vi "Compiled Get Sim Device Settings.vi"(8 "error in (no error)":errorcluster, 9 "Cluster":refnum<k21>, 11 "Addon Ref":T1 format="%.0x") -> (0 "error out":errorcluster, 1 "Async Refs":T2(array[cluster]) {"VS Refs" format="%.0x"}, 2 "Settings":T3[](array[typedef]) {"DTCs"."DM1.Ref"."Data Reference" format="%.0x"; "DTCs"."DM1.Enable.Ref"."Data Reference" format="%.0x"; "DTCs"."DM2.Ref"."Data Reference" format="%.0x"; "DTCs"."DM2.Enable.Ref"."Data Reference" format="%.0x"; "Data"."Outgoing"."Trigger.Refs"."Data Reference" format="%.0x"; "Data"."Outgoing"."Disable.Refs"."Data Reference" format="%.0x"; "Data"."Outgoing"."Data.Refs"."Data Reference" format="%.0x"; "Data"."Incoming"."Timing.Refs"."Data Reference" format="%.0x"; "Data"."Incoming"."Data.Refs"."Data Reference" format="%.0x"; "Network"."Name" format="%.0x"}, 3 "Addon Ref out":T1 format="%.0x")   [LabVIEW 2023, in "J1939 Addon System Explorer.lvlib"]
uses:
  J1939 Addon System Explorer.lvlib
  <vilib>/NI VeriStand/Custom Device API/Custom Device Item Ref.ctl
  Addon Shared/Types/Complied Simulated Device Settings.ctl
  Addon Shared/Types/Monitor Settings.ctl
  Addon Shared/Types/Device Settings.ctl
  Addon Shared/Types/Incoming Settings.ctl
  Addon Shared/Types/Incoming Frame Settings.ctl
  <vilib>/NI VeriStand/Custom Device API/Block Data Reference.ctl
  <vilib>/NI VeriStand/Custom Device API/Data Reference.ctl
  Addon Shared/Types/Outgoing Settings.ctl
  Addon Shared/Types/Outgoing Frame Settings.ctl
  Addon Shared/Types/Outgoing Event Trigger Types.ctl
  SubModules/Frame-Protection-Support/Source/Shared/Types/Exported Frame Settings.ctl
  SubModules/Frame-Protection-Support/Source/Shared/Types/Exported Frame Type.ctl
  SubModules/Frame-Protection-Support/Source/Shared/Types/Exported Protection Settings.ctl
  SubModules/Frame-Protection-Support/Source/Shared/Types/Protection Type.ctl
  SubModules/Frame-Protection-Support/Source/Shared/Types/XNET Signal Configuration.ctl
  SubModules/Frame-Protection-Support/Source/Shared/Types/Exported Counter Settings.ctl
  SubModules/Frame-Protection-Support/Source/Shared/Types/Exported Event Trigger Type.ctl
  Addon Shared/Types/Compiled Simulated Settings.ctl
  Addon Shared/SubVIs/Constants.vi
  <vilib>/NI VeriStand/Custom Device Tools/Custom Device Utility Library/NI VeriStand - Search for All Items by GUID.vi
  <vilib>/NI VeriStand/Custom Device Tools/Custom Device Utility Library/Custom Device Utility Library.lvlib
  Addon Shared/J1939 Addon Shared.lvlib
  <vilib>/NI VeriStand/Custom Device API/Custom Device API.lvlib
  SubModules/Frame-Protection-Support/Source/Shared/Protection and Counter Support Shared.lvlib
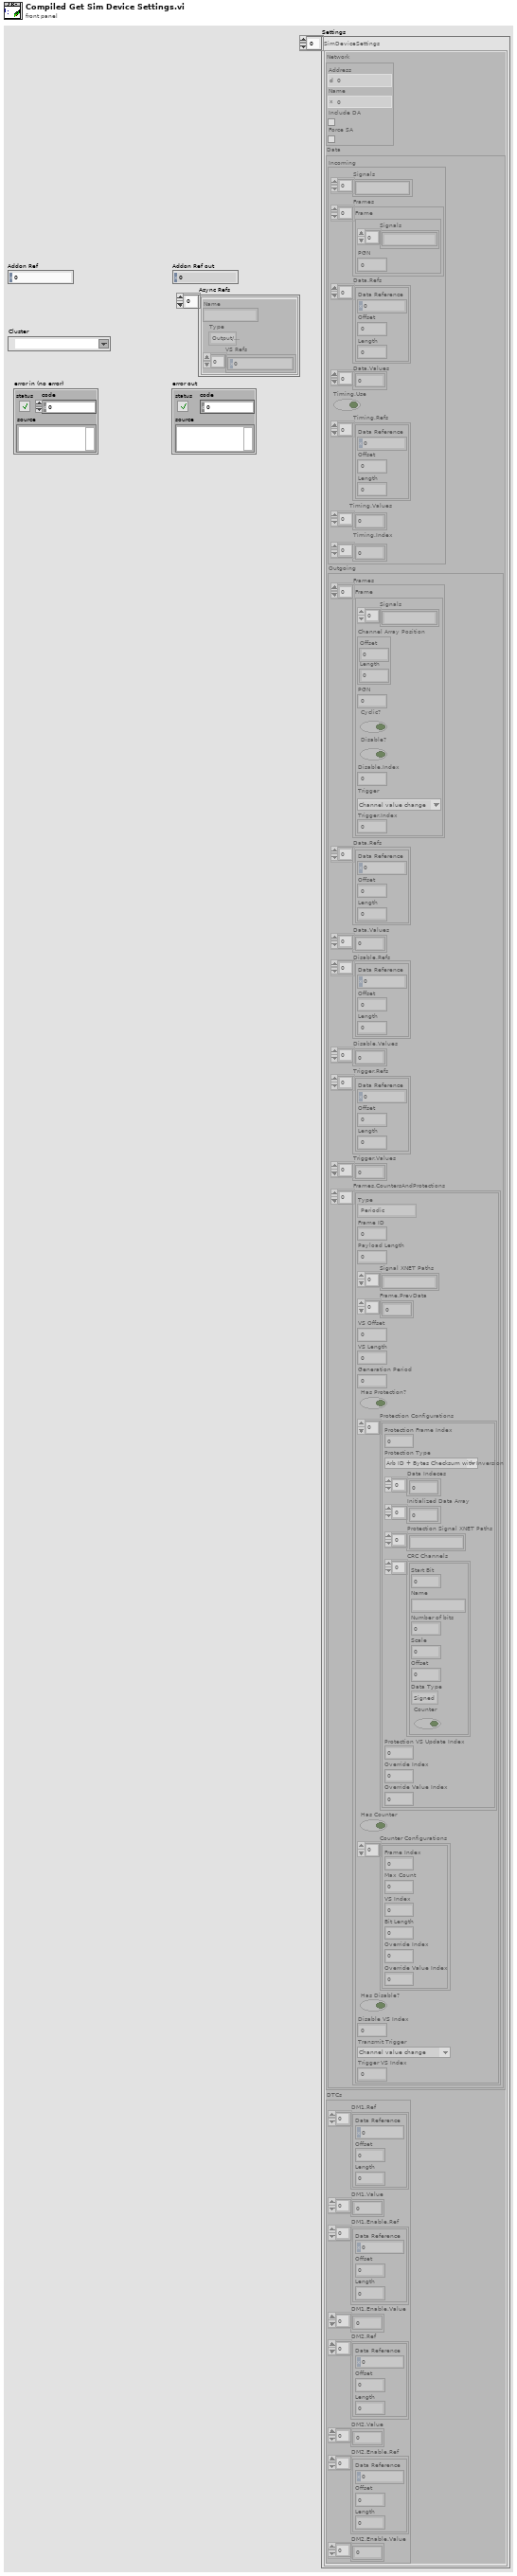
[diagram p1: front panel]
types:
  T1 = typedef "Custom Device API.lvlib/Custom Device Item Ref.ctl" = u64
  T2 = cluster{"Name":string, "Type":enum16{"Output/Write", "Input/Read", "Input/ReadWrite"}, "VS Refs":T1[]}[]
  T3 = typedef "J1939 Addon Shared.lvlib/Complied Simulated Device Settings.ctl" = cluster{"Network":T4, "Data":T5, "DTCs":T20}
  T4 = typedef "J1939 Addon Shared.lvlib/Monitor Settings.ctl" = cluster{"Address":u8, "Name":u64, "Include DA":bool, "Force SA":bool}
  T5 = typedef "J1939 Addon Shared.lvlib/Device Settings.ctl" = cluster{"Incoming":T6, "Outgoing":T10}
  T6 = typedef "J1939 Addon Shared.lvlib/Incoming Settings.ctl" = cluster{"Signals":string[], "Frames":T7[], "Data.Refs":T8[], "Data.Values":dbl[], "Timing.Use":bool, "Timing.Refs":T8[], "Timing.Values":dbl[], "Timing.Index":i32[]}
  T7 = typedef "J1939 Addon Shared.lvlib/Incoming Frame Settings.ctl" = cluster{"Signals":string[], "PGN":u32}
  T8 = typedef "Custom Device API.lvlib/Block Data Reference.ctl" = cluster{"Data Reference":T9, "Offset":u64, "Length":u64}
  T9 = typedef "Custom Device API.lvlib/Data Reference.ctl" = i32
  T10 = typedef "J1939 Addon Shared.lvlib/Outgoing Settings.ctl" = cluster{"Frames":T11[], "Data.Refs":T8[], "Data.Values":dbl[], "Disable.Refs":T8[], "Disable.Values":dbl[], "Trigger.Refs":T8[], "Trigger.Values":dbl[], "Frames.CountersAndProtections":T13[]}
  T11 = typedef "J1939 Addon Shared.lvlib/Outgoing Frame Settings.ctl" = cluster{"Signals":string[], "Channel Array Position":cluster{"Offset":u32, "Length":u32}, "PGN":u32, "Cyclic?":bool, "Disable?":bool, "Disable.Index":i32, "Trigger":T12, "Trigger.Index":i32}
  T12 = typedef "J1939 Addon Shared.lvlib/Outgoing Event Trigger Types.ctl" = enum16{"Channel value change", "Trigger channel (not zero)", "Channel value change or trigger channel (not zero)", "Trigger channel (any value change)", "Channel value change or trigger channel (any value change)"}
  T13 = typedef "Protection and Counter Support Shared.lvlib/Exported Frame Settings.ctl" = cluster{"Type":T14, "Frame ID":u32, "Payload Length":u32, "Signal XNET Paths":string[], "Frame.PrevData":dbl[], "VS Offset":i32, "VS Length":i32, "Generation Period":u32, "Has Protection?":bool, "Protection Configurations":T15[], "Has Counter":bool, "Counter Configurations":T18[], "Has Disable?":bool, "Disable VS Index":i32, "Transmit Trigger":T19, "Trigger VS Index":i32}
  T14 = typedef "Protection and Counter Support Shared.lvlib/Exported Frame Type.ctl" = enum16{"Periodic", "Event", "Periodic/Event"}
  T15 = typedef "Protection and Counter Support Shared.lvlib/Exported Protection Settings.ctl" = cluster{"Protection Frame Index":i32, "Protection Type":T16, "Data Indeces":i32[], "Initialized Data Array":dbl[], "Protection Signal XNET Paths":string[], "CRC Channels":T17[], "Protection VS Update Index":i32, "Override Index":i32, "Override Value Index":i32}
  T16 = typedef "Protection and Counter Support Shared.lvlib/Protection Type.ctl" = enum16{"Arb ID + Bytes Checksum with Inversion", "Arb ID + Bytes CRC with Inversion", "Reversed Raw Signal Checksum with Inversion", "Concatenated Two's Compliment"}
  T17 = typedef "Protection and Counter Support Shared.lvlib/XNET Signal Configuration.ctl" = cluster{"Start Bit":i32, "Name":string, "Number of bits":i32, "Scale":dbl, "Offset":dbl, "Data Type":u32, "Counter":bool}
  T18 = typedef "Protection and Counter Support Shared.lvlib/Exported Counter Settings.ctl" = cluster{"Frame Index":i32, "Max Count":dbl, "VS Index":i32, "Bit Length":i64, "Override Index":i32, "Override Value Index":i32}
  T19 = typedef "Protection and Counter Support Shared.lvlib/Exported Event Trigger Type.ctl" = enum16{"Channel value change", "Trigger channel (not zero)", "Channel value change or trigger channel (not zero)", "Trigger channel (any value change)", "Channel value change or trigger channel (any value change)"}
  T20 = typedef "J1939 Addon Shared.lvlib/Compiled Simulated Settings.ctl" = cluster{"DM1.Ref":T8[], "DM1.Value":dbl[], "DM1.Enable.Ref":T8[], "DM1.Enable.Value":dbl[], "DM2.Ref":T8[], "DM2.Value":dbl[], "DM2.Enable.Ref":T8[], "DM2.Enable.Value":dbl[]}
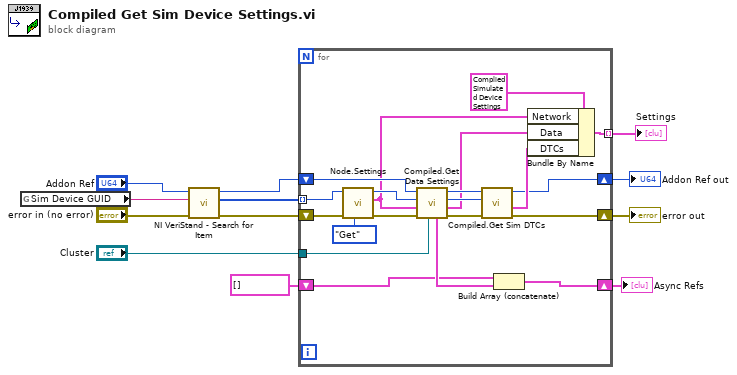
[diagram p0: block diagram]
diagram:
  n1 = global read "Constants.vi" "Sim Device GUID"() -> (w3:string)
  n2 = call-poly <vilib>:"NI VeriStand - Search for Item.vi"("error in"="error in (no error)", "Item GUID"=w3, "Section Ref in"="Addon Ref") -> ("error out"=w5:errorcluster, "Item Refs"=w6:T1[], "Section Ref out"=w9:T1)  [unwired: 5 in, 1 out]
  n3 = for {
    tunnel: w6 -> [w31] mode=indexing
    shift-right: [w19] -> w12
    shift-left: w9 -> [w25]
    shift-right: [w26] -> w10
    shift-left: w5 -> [w32]
    tunnel: "Cluster" -> [w17]
    tunnel: [w28] -> w4 mode=indexing
    shift-right: [w14] -> w1
    shift-left: T2 [] -> [w13]
    n4 = call "Node.Settings.vi"("Action"=enum8{"Get", "Set"}."Get", "error in (no error)"=w32, "Item Ref in"=w31) -> ("error out"=w30:errorcluster, "Node.Settings"=w16:T4, "Item Ref out"=w23:T1)  [unwired: 6 in]
    n5 = call "Compiled.Get Data Settings.vi"("Cluster"=w17, "error in (no error)"=w30, "Node.Settings"=w16, "Node Ref in"=w23, "Addon Ref In"=w25) -> ("error out"=w27:errorcluster, "Node Data Refs"=w21:T5, "Node Ref out"=w22:T1, "Addon Ref out"=w24:T1, "Async Refs"=w15:T2)  [unwired: 2 in]
    n6 = call "Compiled.Get Sim DTCs.vi"("error in (no error)"=w27, "Node Ref in"=w22, "Addon Ref in"=w24) -> ("error out"=w26:errorcluster, "Sim DTCs"=w20:T20, "Addon Ref out"=w19:T1)  [unwired: 5 in, 1 out]
    n7 = Build Array (concatenate)(w13, w15) -> (w14:T2)
    n8 = Bundle By Name(cluster=T3 {"Network"={"Address"=0, "Name"=0, "Include DA"=FALSE, "Force SA"=FALSE}, "Data"={"Incoming"={"Signals"=[], "Frames"=[], "Data.Refs"=[], "Data.Values"=[], "Timing.Use"=FALSE, "Timing.Refs"=[], "Timing.Values"=[], "Timing.Index"=[]}, "Outgoing"={"Frames"=[], "Data.Refs"=[], "Data.Values"=[], "Disable.Refs"=[], "Disable.Values"=[], "Trigger.Refs"=[], "Trigger.Values"=[], "Frames.CountersAndProtections"=[]}}, "DTCs"={"DM1.Ref"=[], "DM1.Value"=[], "DM1.Enable.Ref"=[], "DM1.Enable.Value"=[], "DM2.Ref"=[], "DM2.Value"=[], "DM2.Enable.Ref"=[], "DM2.Enable.Value"=[]}} ("SimDeviceSettings"), "Network"=w16, "Data"=w21, "DTCs"=w20) -> (w28:T3)
  }
  "Addon Ref out" <- w12
  "Settings" <- w4
  "error out" <- w10
  "Async Refs" <- w1
